vi "nanoVoltRead_LightControl.vi"() -> ()   [LabVIEW 2015]
uses:
  <vilib>/Utility/file.llb/Write To Spreadsheet File (string).vi
panel:
  out "Current Run":i32
  in  "Times to Run":i32=1
  in  "Beep when finished":bool=TRUE
  out "error out 2":errorcluster
  out "error out":errorcluster
  in  "Filename Label (optional)":string
  in  "Channel\n(0,1,2)":dbl[](array[numeric])
  out "Light Intensity":dbl
  in  "Event Time\n(s)":dbl[](array[numeric])
  in  "Intensity\n(0-100%)":dbl[](array[numeric])
  in  "Baud Rate":dbl=57600.0
  in  "Light Port":refnum<visa-resource-name>="COM4"
  in  "Previous Top T":dbl
  in  "Temp Rate (s)":dbl=0.25
  in  "Previous Delta T":dbl
  in  "T read time":dbl
  out "Temp2 (C)":dbl format="%#.4g"
  out "Temp1 (C)":dbl format="%#.4g"
  out "Delta T (C)":dbl format="%#.4g"
  in  "Temp2 Port":tag="Dev2"
  in  "Temp1 Port":tag="Dev1"
  in  "Rate (0.1 - 5)":string="5"
  out "Time (s)":dbl caption="Elapsed Time (s)"
  out "XY Graph":cluster{dbl[], dbl[]}[](graph)
  in  "file (use dialog)":path=path "C:/Users/probe_station/Desktop/nanoVolt"
  out "Measurement Number":i32
  in  "stop":bool
  out "Voltage(uV)":dbl
  in  "GPIB\nAddress":string="9"
  # "Keithley Model 2182A Nanovoltmeter Read\n2014-03-19\nMichael Kabatek & David Ellsworth\nCSU Magnetics Lab"
  # "Ignore These"
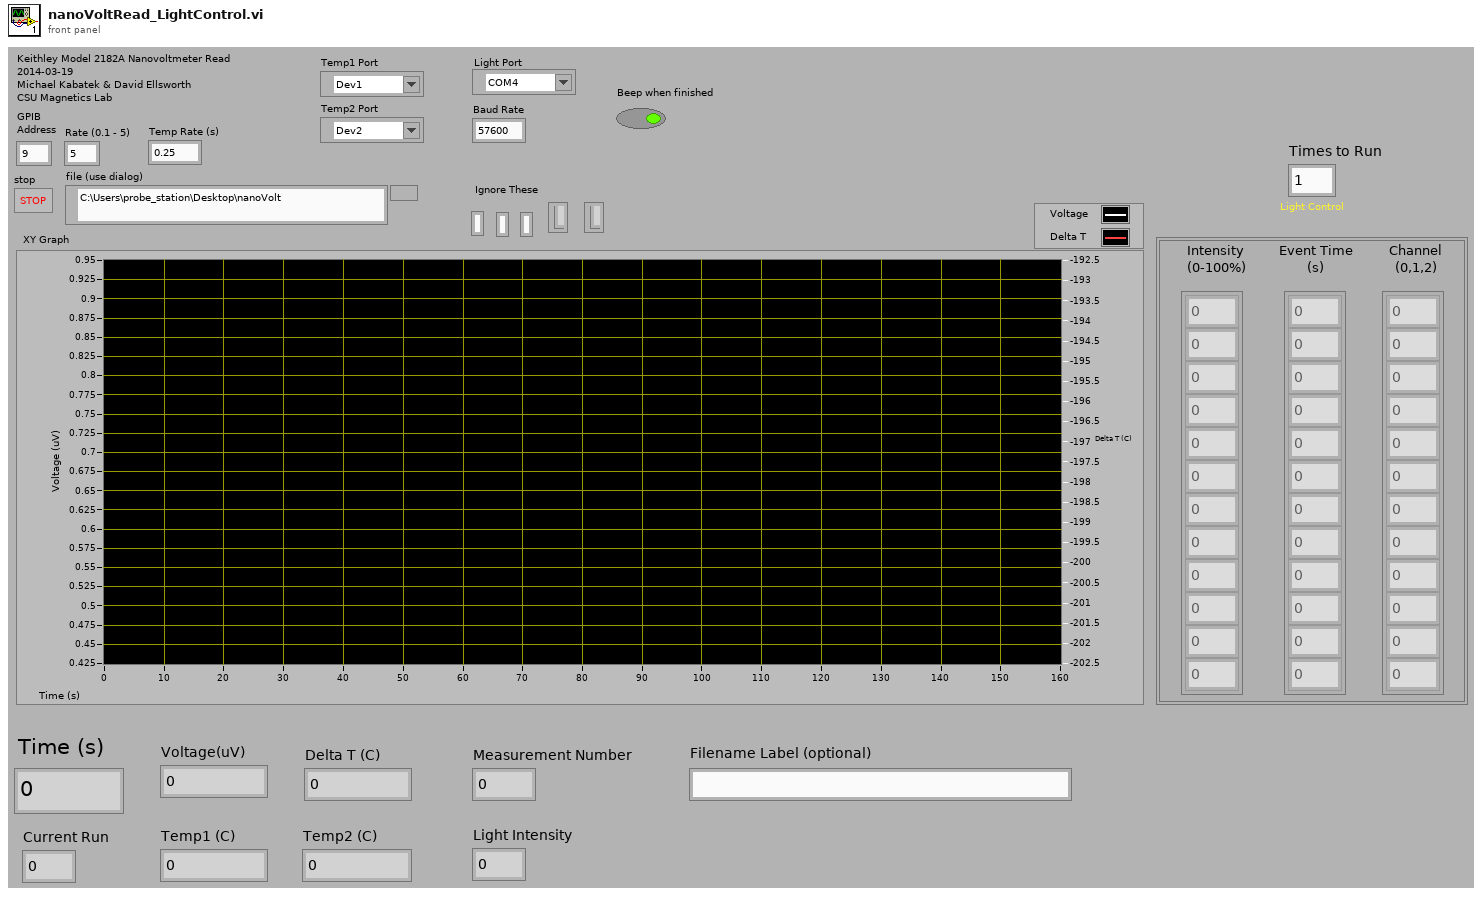
[diagram p1: front panel]
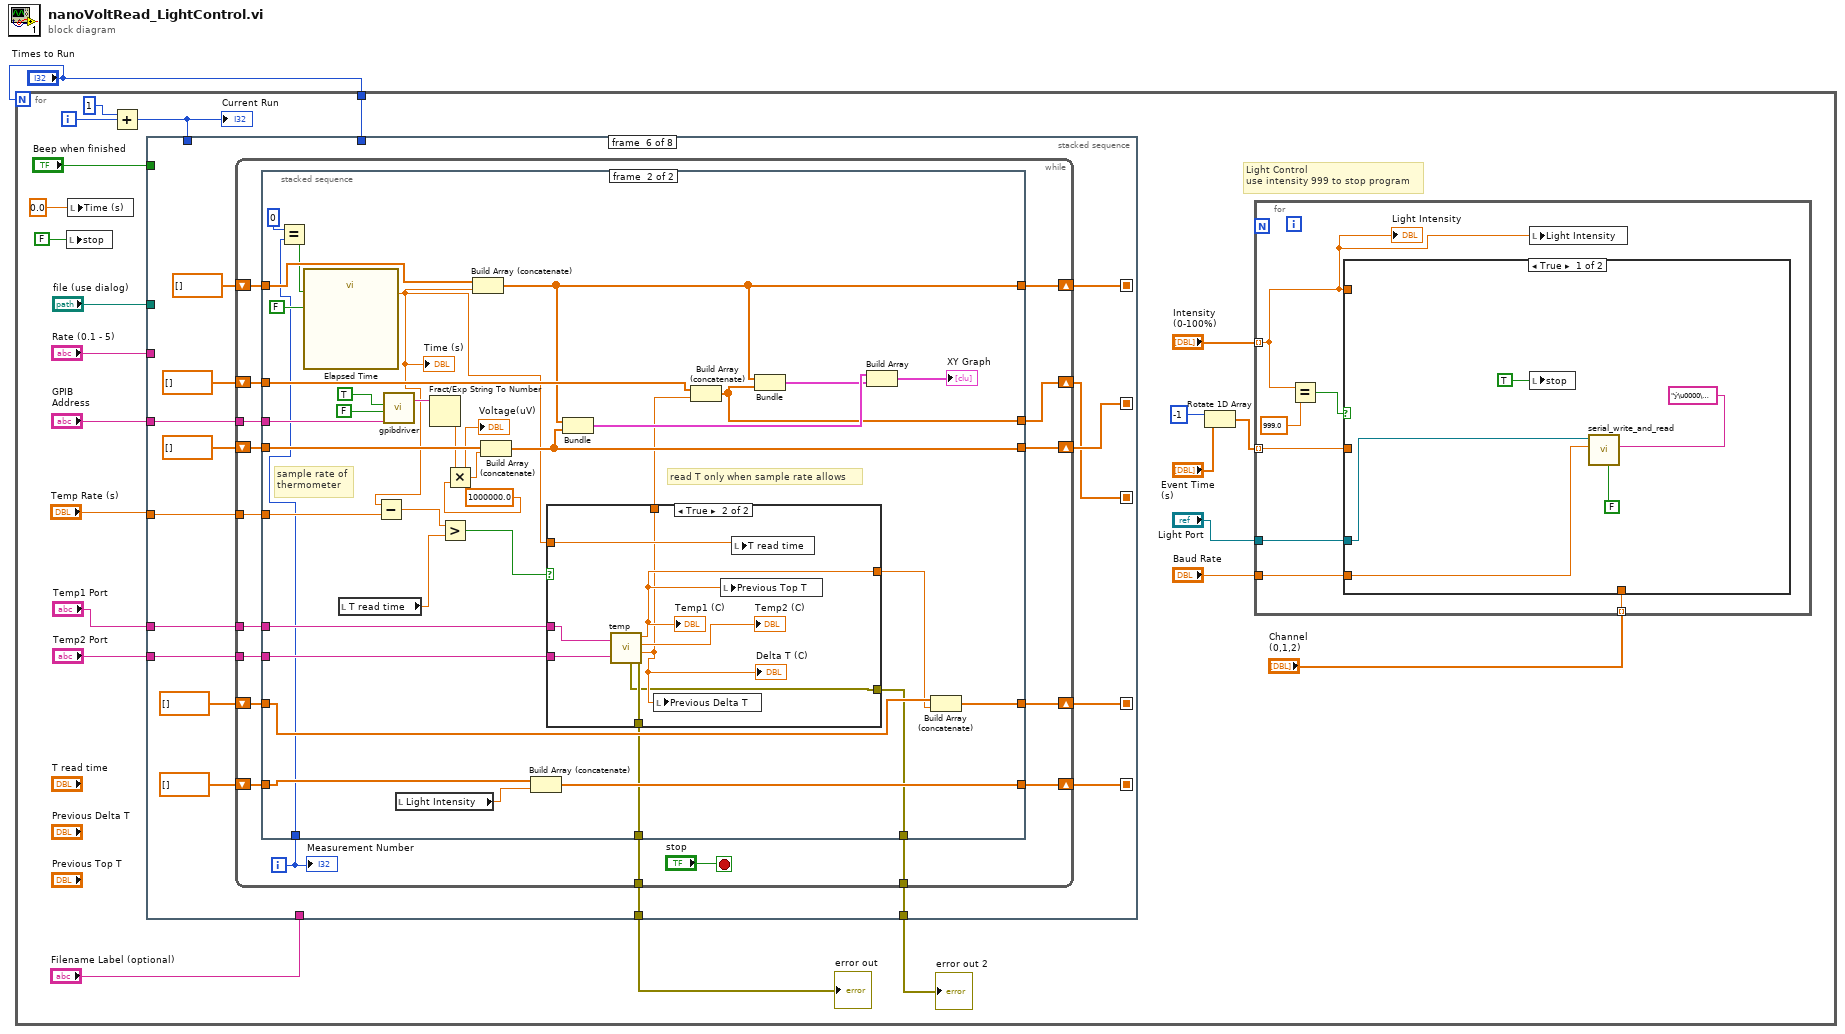
[diagram p0: block diagram]
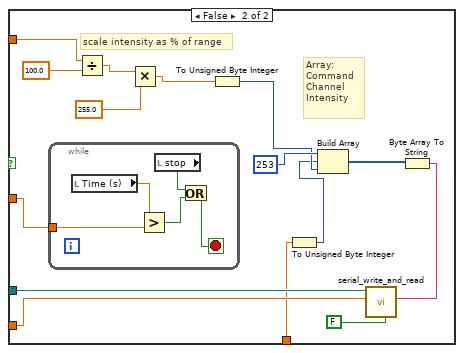
[diagram p2: hidden frame]
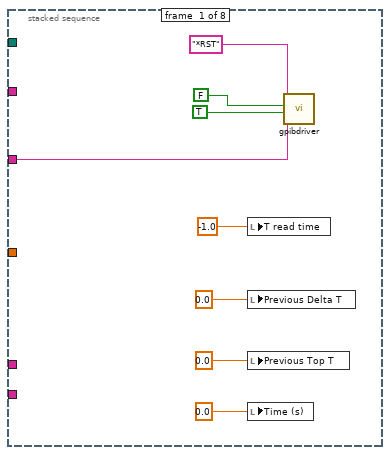
[diagram p3: hidden frame]
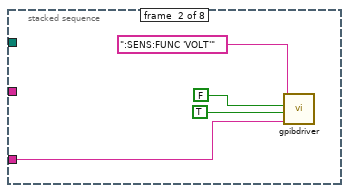
[diagram p4: hidden frame]
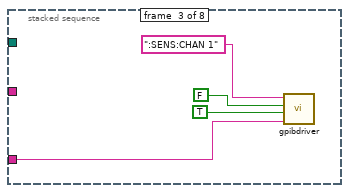
[diagram p5: hidden frame]
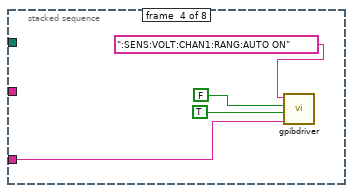
[diagram p6: hidden frame]
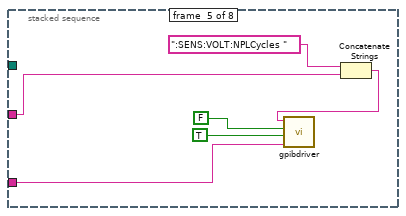
[diagram p7: hidden frame]
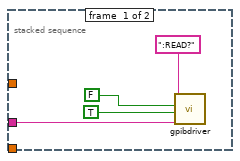
[diagram p8: hidden frame]
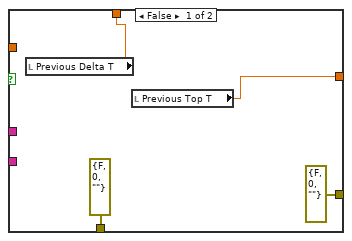
[diagram p9: hidden frame]
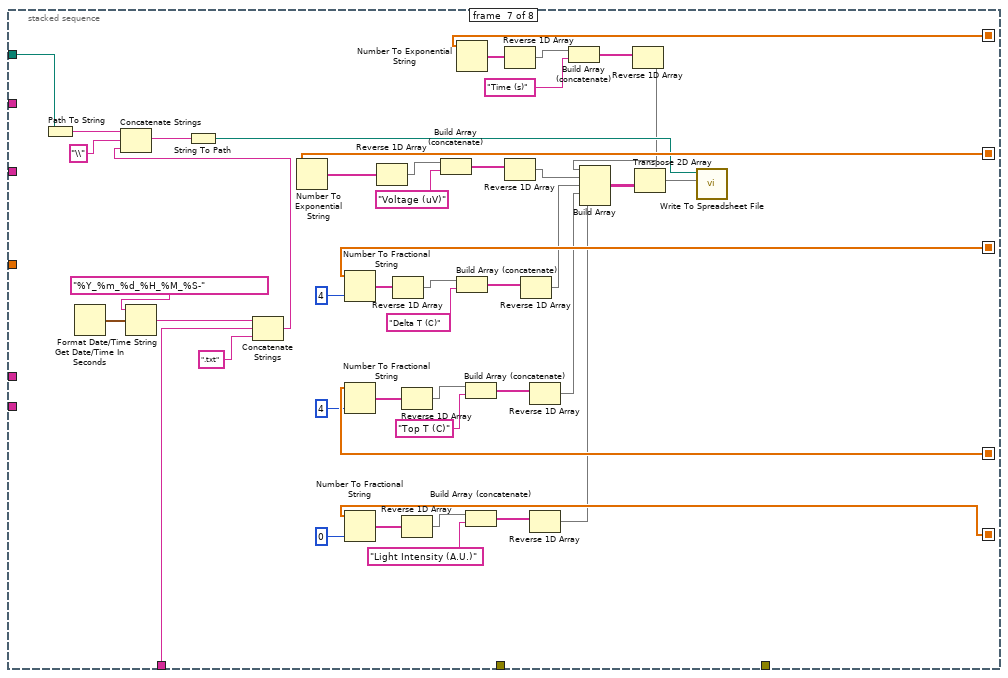
[diagram p10: hidden frame]
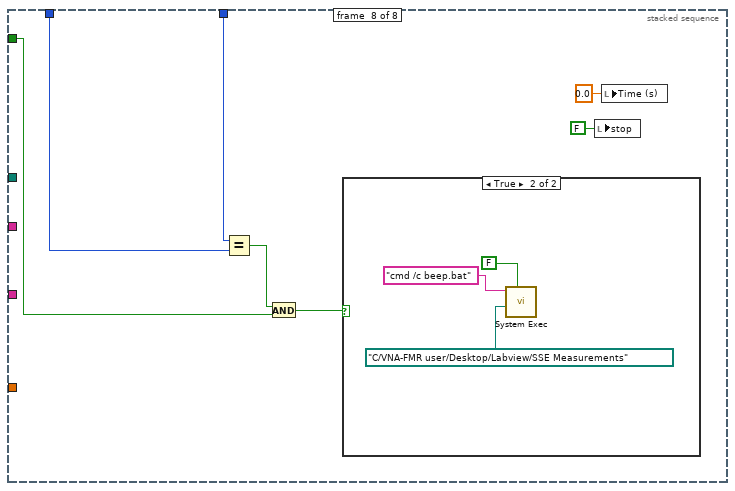
[diagram p11: hidden frame]
diagram:
  n1 = for {
    N: "Times to Run" -> [_]
    tunnel: "Times to Run" -> [w5]
    i -> [w3]
    # "Light Control\nuse intensity 999 to stop program"
    n2 = local write "stop"(FALSE ("stop")) -> ()
    n3 = local write "Time (s)"(0.0 ("Time (s)")) -> ()
    n4 = Add(x=1, y=w3) -> (x+y=w4:i32)
    "Current Run" <- w4
    n5 = stacked-sequence {
      seq-local: [_ _ _ _ _ w96 _ _] -> [_ _ _ _ _ _ w206 _]
      seq-local: [_ _ _ _ _ w94 _ _] -> [_ _ _ _ _ _ w199 _]
      seq-local: [_ _ _ _ _ w91 _ _] -> [_ _ _ _ _ _ w203 _]
      seq-local: [_ _ _ _ _ w88 _ _] -> [_ _ _ _ _ _ w201 _]
      seq-local: [_ _ _ _ _ w85 _ _] -> [_ _ _ _ _ _ w172 _]
      tunnel: "GPIB\nAddress" -> [w61 w65 w69 w73 w80 w98 _ _]
      tunnel: "file (use dialog)" -> [_ _ _ _ _ _ w208 _]
      tunnel: "Temp1 Port" -> [_ _ _ _ _ w93 _ _]
      tunnel: "Temp2 Port" -> [_ _ _ _ _ w92 _ _]
      tunnel: "Rate (0.1 - 5)" -> [_ _ _ _ w77 _ _ _]
      tunnel: "Temp Rate (s)" -> [_ _ _ _ _ w89 _ _]
      tunnel: "Filename Label (optional)" -> [_ _ _ _ _ _ w169 _]
      tunnel: [_ _ _ _ _ w84 _ _] -> w8
      tunnel: [_ _ _ _ _ w83 _ _] -> w7
      tunnel: "Beep when finished" -> [_ _ _ _ _ _ _ w219]
      tunnel: w5 -> [_ _ _ _ _ _ _ w217]
      tunnel: w4 -> [_ _ _ _ _ _ _ w216]
      frame #0 {
        n6 = local write "T read time"(-1.0 ("read T")) -> ()
        n7 = local write "Previous Delta T"(0.0 ("Previous T")) -> ()
        n8 = local write "Previous Top T"(0.0 ("Previous Top T")) -> ()
        n9 = local write "Time (s)"(0.0 ("Time (s)")) -> ()
        n10 = call "gpibdriver.vi"("Characters to Write"="*RST", "Read"=FALSE, "Write"=TRUE ("Write 3"), "GPIB\nAddress"=w61) -> ()  [unwired: 2 in, 1 out]
      }
      frame #1 {
        n11 = call "gpibdriver.vi"("Characters to Write"=":SENS:FUNC 'VOLT'", "Read"=FALSE, "Write"=TRUE ("Write 3"), "GPIB\nAddress"=w65) -> ()  [unwired: 2 in, 1 out]
      }
      frame #2 {
        n12 = call "gpibdriver.vi"("Characters to Write"=":SENS:CHAN 1", "Read"=FALSE, "Write"=TRUE ("Write 3"), "GPIB\nAddress"=w69) -> ()  [unwired: 2 in, 1 out]
      }
      frame #3 {
        n13 = call "gpibdriver.vi"("Characters to Write"=":SENS:VOLT:CHAN1:RANG:AUTO ON", "Read"=FALSE, "Write"=TRUE ("Write 3"), "GPIB\nAddress"=w73) -> ()  [unwired: 2 in, 1 out]
      }
      frame #4 {
        n14 = Concatenate Strings(":SENS:VOLT:NPLCycles " ("Characters to Write"), w77) -> (w78:string)
        n15 = call "gpibdriver.vi"("Characters to Write"=w78, "Read"=FALSE, "Write"=TRUE ("Write 3"), "GPIB\nAddress"=w80) -> ()  [unwired: 2 in, 1 out]
      }
      frame #5 {
        n16 = while {
          tunnel: w98 -> [w116]
          shift-right: [w114] -> w96
          shift-left: dbl[] [] -> [w113]
          shift-right: [w111] -> w94
          shift-left: dbl[] [] -> [w112]
          tunnel: w93 -> [w110]
          tunnel: w92 -> [w109]
          shift-right: [w108] -> w91
          shift-left: dbl[] [] -> [w107]
          tunnel: w89 -> [w106]
          shift-right: [w104] -> w88
          shift-left: dbl[] [] -> [w105]
          shift-right: [w102] -> w85
          shift-left: dbl[] [] -> [w103]
          tunnel: [w101] -> w84
          tunnel: [w100] -> w83
          i -> [w99]
          stop <- "stop" stop-if-true
          n17 = stacked-sequence {
            tunnel: w116 -> [w117 w154]
            tunnel: [_ w149] -> w114
            tunnel: w113 -> [_ w153]
            tunnel: w112 -> [_ w151]
            tunnel: [_ w141] -> w111
            tunnel: w110 -> [_ w148]
            tunnel: w109 -> [_ w147]
            tunnel: [_ w143] -> w108
            tunnel: w107 -> [_ w144]
            tunnel: w106 -> [_ w135]
            tunnel: w105 -> [_ w134]
            tunnel: [_ w132] -> w104
            tunnel: w103 -> [_ w131]
            tunnel: [_ w129] -> w102
            tunnel: [_ w125] -> w101
            tunnel: [_ w124] -> w100
            tunnel: w99 -> [_ w122]
            frame #0 {
              n18 = call "gpibdriver.vi"("Characters to Write"=":READ?", "Read"=FALSE, "Write"=TRUE ("Write 3"), "GPIB\nAddress"=w117) -> ()  [unwired: 2 in, 1 out]
            }
            frame #1 {
              # "read T only when sample rate allows"
              # "sample rate of\nthermometer"
              n19 = Equal?(x=0, y=w122) -> (x = y?=w121:bool)
              n20 = call "Elapsed Time"("Reset"=w121, "Auto Reset"=FALSE) -> ("Elapsed Time (s)"=w138:dbl)  [unwired: 10 in, 7 out]
              "Time (s)" <- w138
              n21 = local read "T read time"() -> (w136:dbl)
              n22 = Subtract(x=w138, y=w135) -> (x-y=w137:dbl)
              n23 = call "gpibdriver.vi"("Read"=TRUE, "Write"=FALSE ("Write 3"), "GPIB\nAddress"=w154) -> ("Characters Read"=w152:string)  [unwired: 3 in]
              n24 = local read "Light Intensity"() -> (w130:dbl)
              n25 = Fract/Exp String To Number(string=w152) -> (number=w128:dbl)  [unwired: 3 in, 1 out]
              n26 = Greater?(x=w137, y=w136) -> (0:w139:bool)
              n27 = Multiply(x=w128, y=1000000.0) -> (x*y=w126:dbl)
              "Voltage(uV)" <- w126
              n28 = Build Array (concatenate)(w151, w138) -> (w141:dbl[])
              n29 = Build Array (concatenate)(w153, w126) -> (w149:dbl[])
              n30 = Build Array (concatenate)(w131, w130) -> (w129:dbl[])
              n31 = case shown="True" w139 {
                tunnel: w148 -> [_ w167]
                tunnel: w147 -> [_ w166]
                tunnel: [w160 w163] -> w145
                tunnel: w138 -> [_ w168]
                tunnel: [w159 w165] -> w133
                tunnel: [errorcluster {"status"=FALSE, "code"=0, "source"=""} ("error out") w162] -> w125
                tunnel: [errorcluster {"status"=FALSE, "code"=0, "source"=""} ("error out 2") w161] -> w124
                frame False {
                  n32 = local read "Previous Delta T"() -> (w160:dbl)
                  n33 = local read "Previous Top T"() -> (w159:dbl)
                }
                frame True {
                  n34 = call "temp.vi"("Temp2 (Bottom) Port"=w166, "Temp1 (Top) Port"=w167) -> ("error out"=w162:errorcluster, "Delta T"=w163:dbl, "Bottom"=→"Temp2 (C)":dbl, "Top"=w165:dbl, "error out 2"=w161:errorcluster)
                  "Delta T (C)" <- w163
                  "Temp1 (C)" <- w165
                  n35 = local write "Previous Delta T"(w163) -> ()
                  n36 = local write "Previous Top T"(w165) -> ()
                  n37 = local write "T read time"(w168) -> ()
                }
              }
              n38 = Bundle(w141, w149) -> (w146:cluster{dbl[], dbl[]})  [unwired: 1 in]
              n39 = Build Array (concatenate)(w144, w145) -> (w143:dbl[])
              n40 = Bundle(w141, w143) -> (w140:cluster{dbl[], dbl[]})  [unwired: 1 in]
              n41 = Build Array(w146, w140) -> (→"XY Graph":cluster{dbl[], dbl[]}[])
              n42 = Build Array (concatenate)(w134, w133) -> (w132:dbl[])
            }
          }
          "Measurement Number" <- w99
        }
      }
      frame #6 {
        n43 = Path To String(path=w208) -> (string=w211:string)
        n44 = Get Date/Time In Seconds() -> (seconds since 1Jan1904=w214:timestamp)
        n45 = Format Date/Time String(time format string (%c)="%Y_%m_%d_%H_%M_%S-", seconds (now)=w214) -> (date/time string=w212:string)  [unwired: 1 in]
        n46 = Concatenate Strings(w212, w169, ".txt" ("string")) -> (w207:string)
        n47 = Concatenate Strings(w211, "\\" ("string"), w207) -> (w209:string)
        n48 = String To Path(string=w209) -> (path=w205:path)
        n49 = Number To Exponential String(number=w206) -> (E-format string=w193:string[])  [unwired: 3 in]
        n50 = Number To Fractional String(number=w203, precision (6)=i16 4) -> (F-format string=w188:string[])  [unwired: 2 in]
        n51 = Number To Fractional String(number=w201, precision (6)=i16 4) -> (F-format string=w181:string[])  [unwired: 2 in]
        n52 = Number To Fractional String(number=w172, precision (6)=i16 0) -> (F-format string=w173:string[])  [unwired: 2 in]
        n53 = Reverse 1D Array(array=w193) -> (reversed array=w192:string[])
        n54 = Reverse 1D Array(array=w188) -> (reversed array=w187:string[])
        n55 = Reverse 1D Array(array=w181) -> (reversed array=w183:string[])
        n56 = Reverse 1D Array(array=w173) -> (reversed array=w175:string[])
        n57 = Build Array (concatenate)(w192, "Voltage (uV)") -> (w191:string[])
        n58 = Number To Exponential String(number=w199) -> (E-format string=w197:string[])  [unwired: 3 in]
        n59 = Build Array (concatenate)(w187, "Delta T (C)") -> (w189:string[])
        n60 = Build Array (concatenate)(w183, "Top T (C)") -> (w184:string[])
        n61 = Build Array (concatenate)(w175, "Light Intensity (A.U.)") -> (w176:string[])
        n62 = Reverse 1D Array(array=w197) -> (reversed array=w196:string[])
        n63 = Reverse 1D Array(array=w191) -> (reversed array=w190:string[])
        n64 = Reverse 1D Array(array=w189) -> (reversed array=w186:string[])
        n65 = Reverse 1D Array(array=w184) -> (reversed array=w180:string[])
        n66 = Reverse 1D Array(array=w176) -> (reversed array=w171:string[])
        n67 = Build Array (concatenate)(w196, "Time (s)") -> (w195:string[])
        n68 = Reverse 1D Array(array=w195) -> (reversed array=w194:string[])
        n69 = Build Array(w194, w190, w186, w180, w171) -> (w198:string[][])
        n70 = Transpose 2D Array(2D array=w198) -> (transposed array=w204:string[][])
        n71 = call-poly <vilib>:"Write To Spreadsheet File.vi"("2D data"=w204, "file path (dialog if empty)"=w205) -> ()  [unwired: 6 in, 1 out]
      }
      frame #7 {
        n72 = Equal?(x=w217, y=w216) -> (x = y?=w215:bool)
        n73 = And(x=w215, y=w219) -> (x .and. y?=w218:bool)
        n74 = case shown="True" w218 {
          frame False {
          }
          frame True {
            n75 = call <vilib>:"System Exec.vi"("wait until completion? (T)"=FALSE, "working directory"=path "C:/VNA-FMR user/Desktop/Labview/SSE Measurements", "command line"="cmd /c beep.bat") -> ()  [unwired: 5 in, 4 out]
          }
        }
        n76 = local write "stop"(FALSE ("stop")) -> ()
        n77 = local write "Time (s)"(0.0 ("Time (s)")) -> ()
      }
    }
    "error out" <- w8
    "error out 2" <- w7
    n78 = Rotate 1D Array(1:"Event Time\n(s)", 2:-1 ("n")) -> (0:w11:dbl[])
    n79 = for {
      tunnel: "Intensity\n(0-100%)" -> [w25] mode=indexing
      tunnel: w11 -> [w29] mode=indexing
      tunnel: "Light Port" -> [w31]
      tunnel: "Baud Rate" -> [w30]
      tunnel: "Channel\n(0,1,2)" -> [w26] mode=indexing
      n80 = Equal?(x=w25, y=999.0) -> (x = y?=w28:bool)
      n81 = case shown="True" w28 {
        tunnel: w31 -> [w35 w43]
        tunnel: w30 -> [w34 w42]
        tunnel: w29 -> [_ w41]
        tunnel: w25 -> [_ w40]
        tunnel: w26 -> [_ w38]
        frame True {
          n82 = local write "stop"(TRUE ("stop")) -> ()
          n83 = call "serial_write_and_read.vi"("VISA resource name"=w35, "baud rate"=w34, "read"=FALSE, "string to write"="ý\u0000\u0000") -> ()  [unwired: 6 in, 1 out]
        }
        frame False {
          # "Array:\nCommand\nChannel\nIntensity"
          # "scale intensity as % of range"
          n84 = while {
            tunnel: w41 -> [w53]
            stop <- w56 stop-if-true
            n85 = local read "Time (s)"() -> (w54:dbl)
            n86 = Greater?(x=w54, y=w53) -> (0:w52:bool)
            n87 = local read "stop"() -> (w55:bool)
            n88 = Or(x=w55, y=w52) -> (x .or. y?=w56:bool)
          }
          n89 = Divide(x=w40, y=100.0) -> (x/y=w50:dbl)
          n90 = Multiply(x=w50, y=255.0) -> (x*y=w48:dbl)
          n91 = To Unsigned Byte Integer(number=w48) -> (unsigned 8bit integer=w39:u8)
          n92 = To Unsigned Byte Integer(number=w38) -> (unsigned 8bit integer=w37:u8)
          n93 = Build Array(u8 253 ("element"), w37, w39) -> (w46:u8[])
          n94 = Byte Array To String(unsigned byte array=w46) -> (string=w45:string)
          n95 = call "serial_write_and_read.vi"("VISA resource name"=w43, "baud rate"=w42, "read"=FALSE, "string to write"=w45) -> ()  [unwired: 6 in, 1 out]
        }
      }
      n96 = local write "Light Intensity"(w25) -> ()
      "Light Intensity" <- w25
    }
  }
